vi "PSVCH_Delete Duplication And Null In Array.vi"(8 "Error In (no error)":errorcluster, 11 "ArrayIn":string[](array[string])) -> (0 "Error Out":errorcluster, 3 "ArrayOut":string[](array[string]))   [LabVIEW 2016]
panel:
  # "Data In"
  # "Data Out"
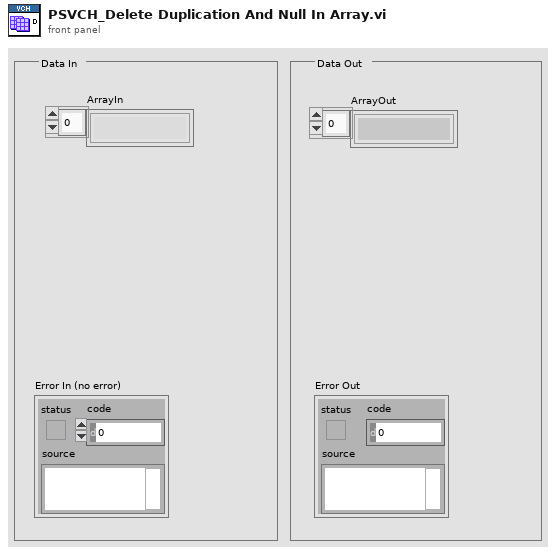
[diagram p1: front panel]
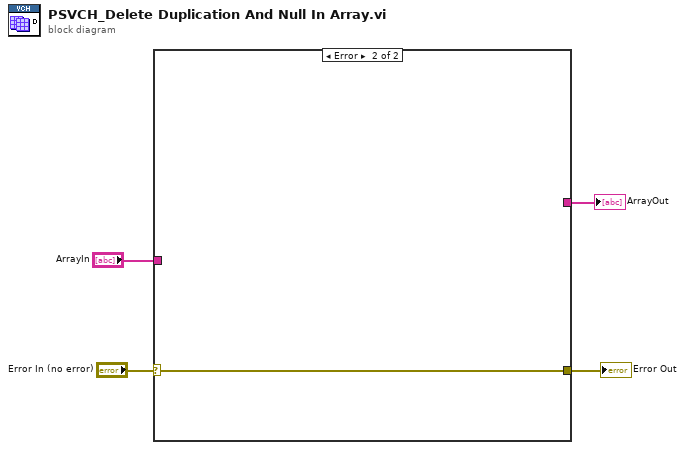
[diagram p0: block diagram]
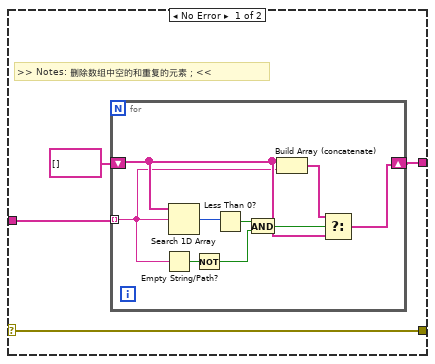
[diagram p2: hidden frame]
diagram:
  n1 = case shown="Error" "Error In (no error)" {
    selector: "Error In (no error)" -> [w5 w18]
    tunnel: [w8 _] -> w4
    tunnel: "ArrayIn" -> [w7 _]
    tunnel: [w5 w18] -> w1
    frame No Error {
      # ">> Notes: 删除数组中空的和重复的元素；<<"
      n2 = for {
        tunnel: w7 -> [w13] mode=indexing
        shift-right: [w14] -> w8
        shift-left: string[] [] -> [w16]
        n3 = Empty String/Path?(string/path=w13) -> (empty?=w11:bool)
        n4 = Search 1D Array(1D array=w16, element=w13) -> (index of element=w17:i32)  [unwired: 1 in]
        n5 = Not(x=w11) -> (.not. x?=w10:bool)
        n6 = Less Than 0?(x=w17) -> (x < 0?=w12:bool)
        n7 = And(x=w12, y=w10) -> (x .and. y?=w9:bool)
        n8 = Build Array (concatenate)(w16, w13) -> (w15:string[])
        n9 = Select(t=w15, s=w9, f=w16) -> (s? t:f=w14:string[])
      }
    }
    frame Error {
    }
  }
  "ArrayOut" <- w4
  "Error Out" <- w1
